vi "readScriptCommandLine.vi"(8 "error in (no error)":errorcluster, 11 "Enter Line Number":u32=2) -> (0 "error out":errorcluster, 3 "standard output":string="2. ; Script for testing ASIC and pin driver hardware                        \t\t\r\n\r\n")   [LabVIEW 2015]
panel:
  out "standard error":string
  out "return code":i32
  in  "command line":string="py -3 readScript.py "
  in  "working directory":path=path "C:/modisEdge/Scanner/Test Sequence/TestScripts"
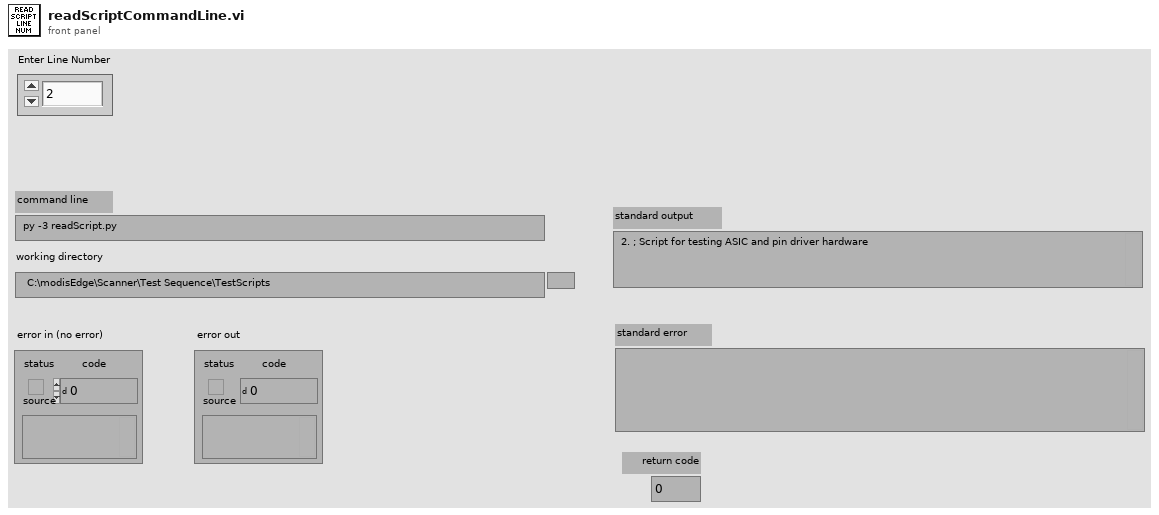
[diagram p1: front panel]
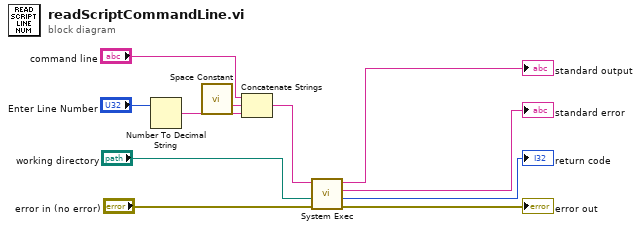
[diagram p0: block diagram]
diagram:
  n1 = Number To Decimal String(number="Enter Line Number") -> (decimal integer string=w4:string)  [unwired: 1 in]
  n2 = call <vilib>:"Space Constant.vi"() -> ("String"=w5:string)
  n3 = Concatenate Strings("command line", w5, w4) -> (w1:string)
  n4 = call <vilib>:"System Exec.vi"("error in (no error)"="error in (no error)", "working directory"="working directory", "command line"=w1) -> ("error out"=→"error out":errorcluster, "return code"=→"return code":i32, "standard error"=→"standard error":string, "standard output"=→"standard output":string)  [unwired: 5 in]
